vi "Initialize Acquisition Data.vi"(8 "error in (no error)":errorcluster, 10 "Channel Mask":u64, 11 "DriverMasterSync in":refnum<class "DriverMasterSync.lvclass">) -> (0 "error out":errorcluster, 3 "DriverMasterSync out":refnum<class "DriverMasterSync.lvclass">)   [LabVIEW 2014, in "DriverMasterSync.lvlib" / "DriverMasterSync.lvclass"]
uses:
  DriverMasterSync.lvclass
  DriverMasterSync.lvclass/DriverMasterSync.ctl
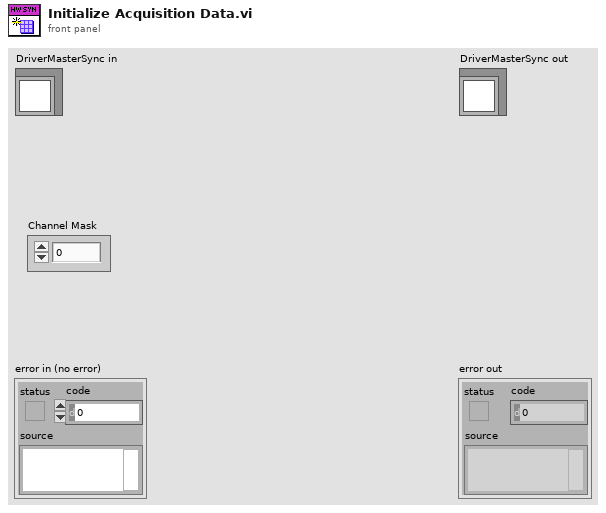
[diagram p1: front panel]
types:
  T1 = typedef "WINFAS 2 Data Queue.lvlib/Acquisition Data Cluster.ctl" = T2[]
  T2 = typedef "WINFAS 2 Data Queue.lvlib/Acquisition Data 1 Sample Cluster.ctl" = cluster{"TDX":sgl[], "Encoder":sgl}
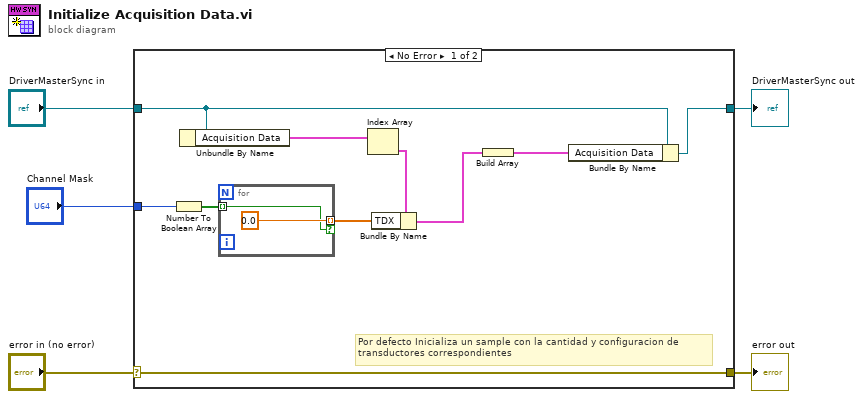
[diagram p0: block diagram]
diagram:
  n1 = case shown="No Error" "error in (no error)" {
    selector: "error in (no error)" -> [w15 w19]
    tunnel: [w15 w19] -> w4
    tunnel: [w6 w18] -> w2
    tunnel: "DriverMasterSync in" -> [w7 w18]
    tunnel: "Channel Mask" -> [w13 _]
    frame No Error {
      # "Por defecto Inicializa un sample con la cantidad y configuracion de\ntransductores correspondientes"
      n2 = Number To Boolean Array(number=w13) -> (Boolean array=w14:bool[])
      n3 = Unbundle By Name(w7) -> ("Acquisition Data"=w12:T1)
      n4 = for {
        tunnel: w14 -> [w16] mode=indexing
        tunnel: [sgl 0.0] -> w10 mode=indexing if=w16
      }
      n5 = Index Array(array=w12) -> (element=w11:T2)  [unwired: 1 in]
      n6 = Bundle By Name(cluster=w11, "TDX"=w10) -> (w9:T2)
      n7 = Build Array(w9) -> (w8:T2[])
      n8 = Bundle By Name(cluster=w7, "Acquisition Data"=w8) -> (w6:refnum<class "DriverMasterSync.lvclass">)
    }
    frame Error {
    }
  }
  "error out" <- w4
  "DriverMasterSync out" <- w2
